vi "fichero.vi"(8 "error in (no error)":errorcluster, 9 "Formato":string, 10 "Nombre":string, 11 "Direccion":path) -> (0 "error out":errorcluster, 3 "Byte Stream File out":refnum<file>)   [LabVIEW 2020]
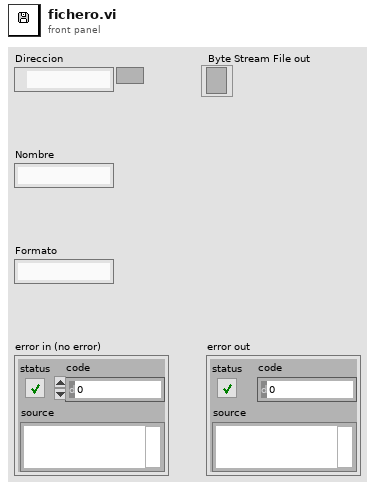
[diagram p1: front panel]
types:
  T1 = enum16{"open", "replace", "create", "open or create", "replace or create", "replace or create with confirmation"}
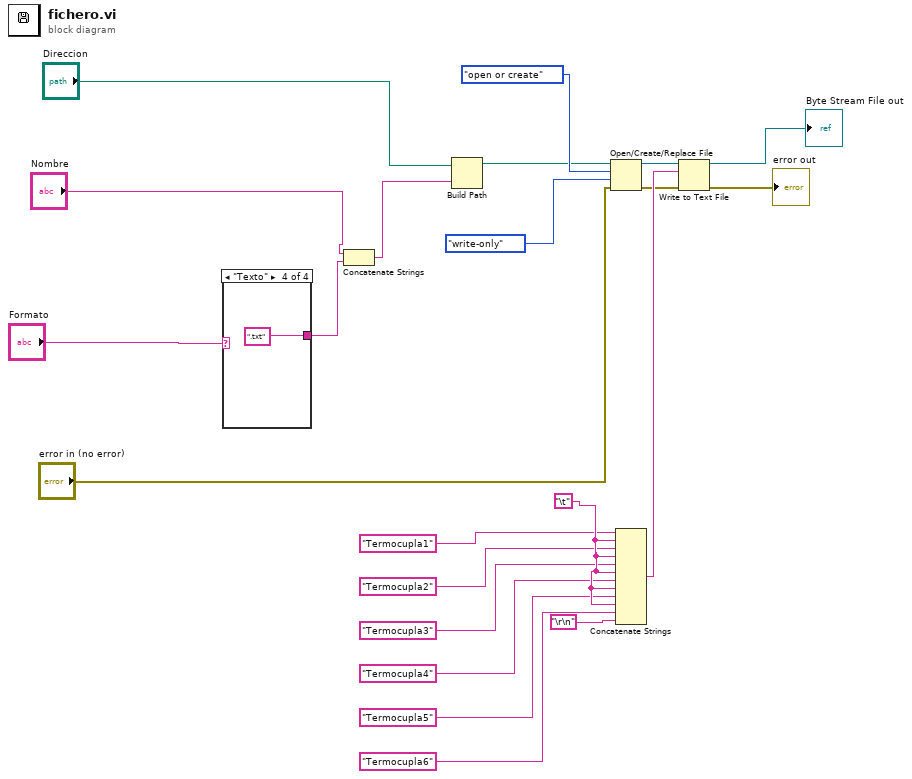
[diagram p0: block diagram]
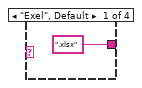
[diagram p2: hidden frame]
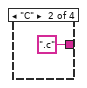
[diagram p3: hidden frame]
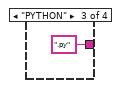
[diagram p4: hidden frame]
diagram:
  w16 = "\t"
  n1 = case shown="\"Texto\"" "Formato" {
    tunnel: [".xlsx" ".c" ".py" ".txt"] -> w4
    frame "Exel", Default {
    }
    frame "C" {
    }
    frame "PYTHON" {
    }
    frame "Texto" {
    }
  }
  n2 = Concatenate Strings("Nombre", w4) -> (w5:string)
  n3 = Build Path(base path="Direccion", name or relative path=w5) -> (appended path=w6:path)
  n4 = Open/Create/Replace File(file path (use dialog)=w6, error in="error in (no error)", operation (0:open)=T1."open or create", access (0:read/write)=enum16{"read/write", "read-only", "write-only"}."write-only") -> (refnum out=w18:refnum<file>, error out=w19:errorcluster)  [unwired: 2 in, 1 out]
  n5 = Concatenate Strings("Termocupla1", w16, "Termocupla2", w16, "Termocupla3", w16, "Termocupla4", w16, "Termocupla5", w16, "Termocupla6", "\r\n") -> (w20:string)
  n6 = Write to Text File(file (use dialog)=w18, text=w20, error in=w19) -> (refnum out=→"Byte Stream File out":refnum<file>, error out=→"error out":errorcluster)  [unwired: 1 in, 1 out]
